vi "Delete In Folder.vi"(8 "error in (no error)":errorcluster, 10 "ProjectItem in":refnum<vi>) -> (0 "error out":errorcluster)   [LabVIEW 2019]
uses:
  gRPC Template Creation Utility.lvlib
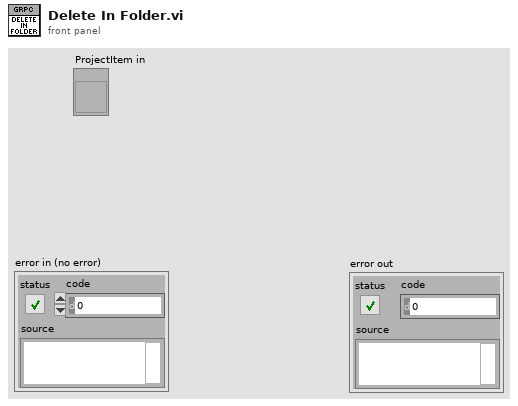
[diagram p1: front panel]
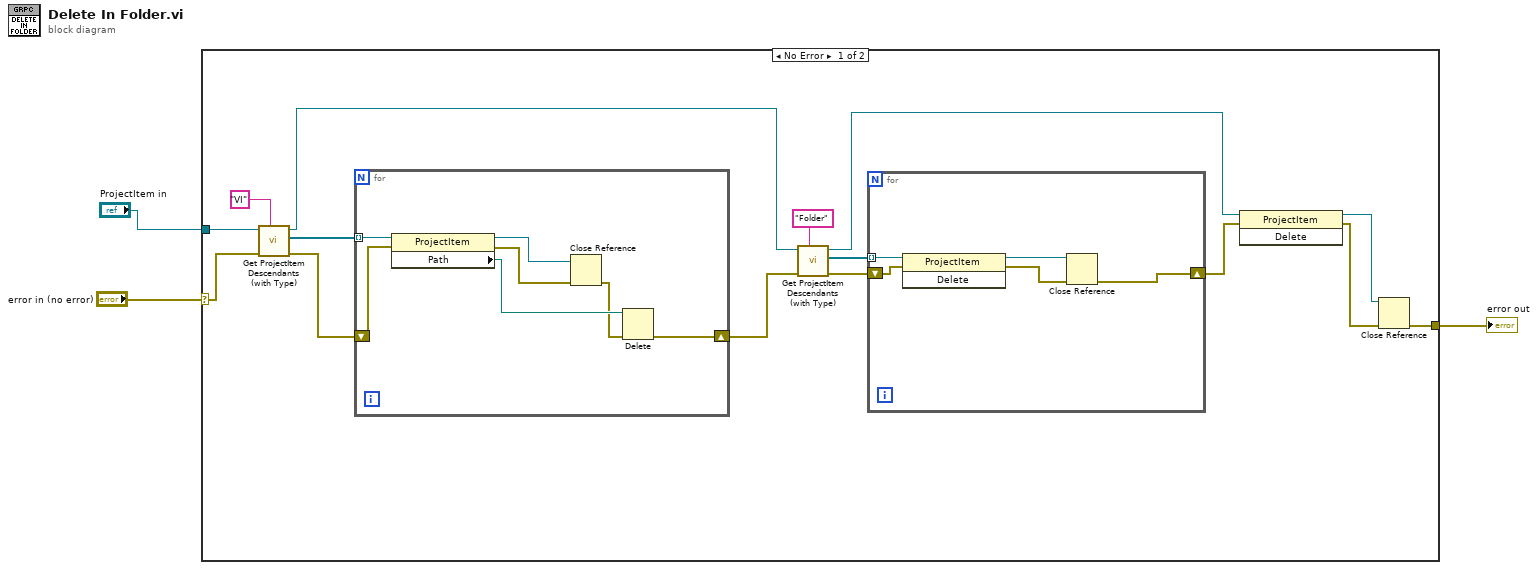
[diagram p0: block diagram]
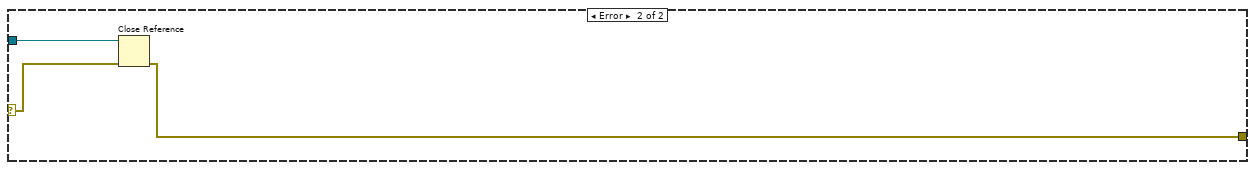
[diagram p2: hidden frame]
diagram:
  n1 = case shown="No Error" "error in (no error)" {
    selector: "error in (no error)" -> [w5 w32]
    tunnel: "ProjectItem in" -> [w18 w33]
    tunnel: [w6 w31] -> w1
    frame No Error {
      n2 = call "Get ProjectItem Descendants (with Type).vi"("Type"="VI", "error in (no error)"=w5, "ProjectItem in"=w18) -> ("error out"=w4:errorcluster, "All Descendents"=w16:refnum<vi>[], "ProjectItem out"=w15:refnum<vi>)  [unwired: 6 in]
      n3 = for {
        tunnel: w16 -> [w30] mode=indexing
        shift-right: [w24] -> w12
        shift-left: w4 -> [w27]
        n4 = property class="ProjectItem"(reference=w30, error in=w27) -> (reference out=w29:refnum<vi>, error out=w26:errorcluster, "Path"=w28:path)
        n5 = Close Reference(reference=w29, error in (no error)=w26) -> (error out=w25:errorcluster)
        n6 = Delete(path (use dialog)=w28, error in=w25) -> (error out=w24:errorcluster)  [unwired: 3 in, 2 out]
      }
      n7 = call "Get ProjectItem Descendants (with Type).vi"("Type"="Folder", "error in (no error)"=w12, "ProjectItem in"=w15) -> ("error out"=w11:errorcluster, "All Descendents"=w13:refnum<vi>[], "ProjectItem out"=w10:refnum<vi>)  [unwired: 6 in]
      n8 = for {
        tunnel: w13 -> [w23] mode=indexing
        shift-right: [w19] -> w8
        shift-left: w11 -> [w21]
        n9 = invoke class="ProjectItem" method="Delete"(reference=w23, error in=w21) -> (reference out=w22:refnum<vi>, error out=w20:errorcluster)  [unwired: 1 in, 1 out]
        n10 = Close Reference(reference=w22, error in (no error)=w20) -> (error out=w19:errorcluster)
      }
      n11 = invoke class="ProjectItem" method="Delete"(reference=w10, error in=w8) -> (reference out=w9:refnum<vi>, error out=w7:errorcluster)  [unwired: 1 in, 1 out]
      n12 = Close Reference(reference=w9, error in (no error)=w7) -> (error out=w6:errorcluster)
    }
    frame Error {
      n13 = Close Reference(reference=w33, error in (no error)=w32) -> (error out=w31:errorcluster)
    }
  }
  "error out" <- w1
